vi "Untitled 2.vi"() -> ()   [LabVIEW 2014]
uses:
  Global 1.vi
panel:
  out "String":string
  in  "?":T1
  # "by Siavash Aghajani"
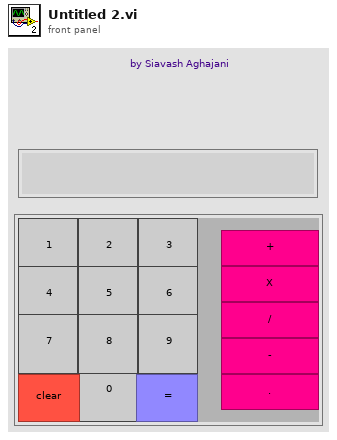
[diagram p1: front panel]
types:
  T1 = cluster{"Blank Button 2":bool, "Blank Button 3":bool, "Blank Button 4":bool, "Blank Button 5":bool, "Blank Button 6":bool, "Blank Button 7":bool, "Blank Button 8":bool, "Blank Button 9":bool, "Blank Button 10":bool, "Blank Button":bool, "Blank Button 11":bool, "Blank Button 12":bool, "Blank Button 13":bool, "Blank Button 14":bool, "Blank Button 15":bool, "Blank Button 16":bool, "OK Button":bool}
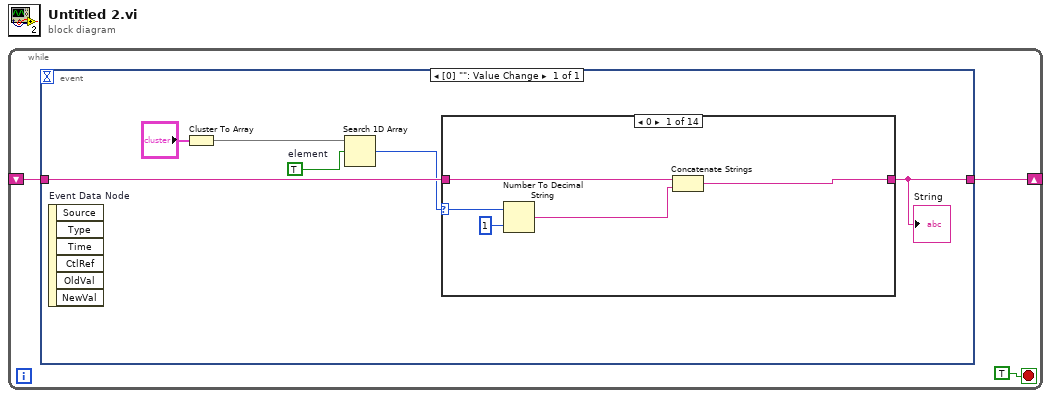
[diagram p0: block diagram]
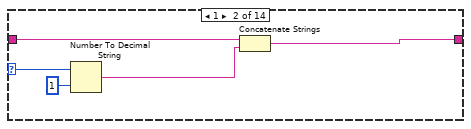
[diagram p2: hidden frame]
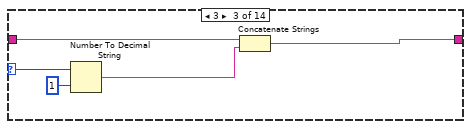
[diagram p3: hidden frame]
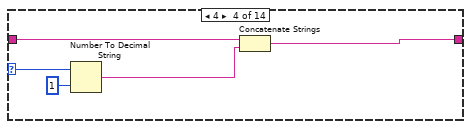
[diagram p4: hidden frame]
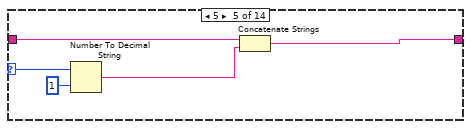
[diagram p5: hidden frame]
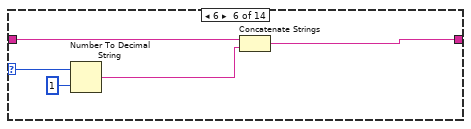
[diagram p6: hidden frame]
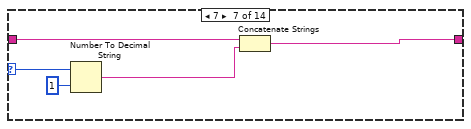
[diagram p7: hidden frame]
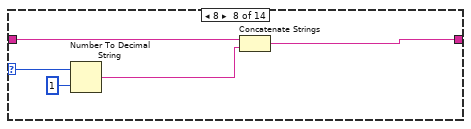
[diagram p8: hidden frame]
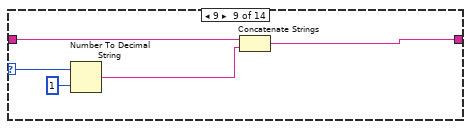
[diagram p9: hidden frame]
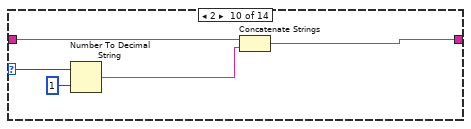
[diagram p10: hidden frame]
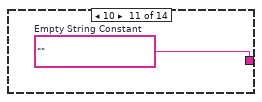
[diagram p11: hidden frame]
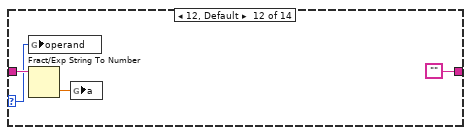
[diagram p12: hidden frame]
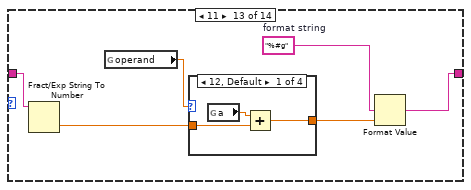
[diagram p13: hidden frame]
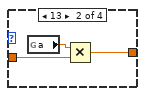
[diagram p14: hidden frame]
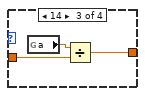
[diagram p15: hidden frame]
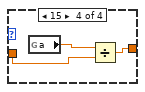
[diagram p16: hidden frame]
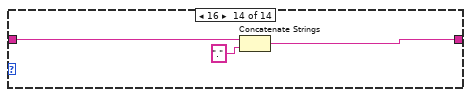
[diagram p17: hidden frame]
diagram:
  n1 = while {
    shift-right: [w1] -> _
    shift-left: _ -> [w2]
    stop <- TRUE stop-if-true
    n2 = event shown="[0] \"\": Value Change" {
      selector: _ -> [_]
      dyn-events: _ -> [_]
      timeout: _ -> [_]
      tunnel: w2 -> [w6]
      tunnel: [w5] -> w1
      event Value Change {
        w7 = TRUE  # element
        n3 = event-data "Event Data Node"() -> ()  [unwired: 1 in, 6 out]
        n4 = Cluster To Array(cluster="?") -> (array=w9:bool[])
        n5 = Search 1D Array(1D array=w9, element=w7) -> (index of element=w4:i32)  [unwired: 1 in]
        n6 = case shown="0" w4 {
          selector: w4 -> [w11 w16 w21 w26 w31 w36 w41 w46 w51 w56 _ w62 _ _]
          tunnel: w6 -> [w13 w18 w23 w28 w33 w38 w43 w48 w53 w58 _ w64 w69 w84]
          tunnel: [w12 w17 w22 w27 w32 w37 w42 w47 w52 w57 w60 "" w66 w85] -> w5
          frame 0 {
            n7 = Number To Decimal String(number=w11, width (-)=i16 1) -> (decimal integer string=w14:string)
            n8 = Concatenate Strings "Concatenate Strings"(w13, w14) -> (w12:string)
          }
          frame 1 {
            n9 = Number To Decimal String(number=w16, width (-)=i16 1) -> (decimal integer string=w19:string)
            n10 = Concatenate Strings "Concatenate Strings"(w18, w19) -> (w17:string)
          }
          frame 3 {
            n11 = Number To Decimal String(number=w21, width (-)=i16 1) -> (decimal integer string=w24:string)
            n12 = Concatenate Strings "Concatenate Strings"(w23, w24) -> (w22:string)
          }
          frame 4 {
            n13 = Number To Decimal String(number=w26, width (-)=i16 1) -> (decimal integer string=w29:string)
            n14 = Concatenate Strings "Concatenate Strings"(w28, w29) -> (w27:string)
          }
          frame 5 {
            n15 = Number To Decimal String(number=w31, width (-)=i16 1) -> (decimal integer string=w34:string)
            n16 = Concatenate Strings "Concatenate Strings"(w33, w34) -> (w32:string)
          }
          frame 6 {
            n17 = Number To Decimal String(number=w36, width (-)=i16 1) -> (decimal integer string=w39:string)
            n18 = Concatenate Strings "Concatenate Strings"(w38, w39) -> (w37:string)
          }
          frame 7 {
            n19 = Number To Decimal String(number=w41, width (-)=i16 1) -> (decimal integer string=w44:string)
            n20 = Concatenate Strings "Concatenate Strings"(w43, w44) -> (w42:string)
          }
          frame 8 {
            n21 = Number To Decimal String(number=w46, width (-)=i16 1) -> (decimal integer string=w49:string)
            n22 = Concatenate Strings "Concatenate Strings"(w48, w49) -> (w47:string)
          }
          frame 9 {
            n23 = Number To Decimal String(number=w51, width (-)=i16 1) -> (decimal integer string=w54:string)
            n24 = Concatenate Strings "Concatenate Strings"(w53, w54) -> (w52:string)
          }
          frame 2 {
            n25 = Number To Decimal String(number=w56, width (-)=i16 1) -> (decimal integer string=w59:string)
            n26 = Concatenate Strings "Concatenate Strings"(w58, w59) -> (w57:string)
          }
          frame 10 {
            w60 = ""  # Empty String Constant
          }
          frame 12, Default {
            n27 = global write "Global 1.vi" "operand"(w62) -> ()
            n28 = Fract/Exp String To Number(string=w64) -> (number=w61:dbl)  [unwired: 3 in, 1 out]
            n29 = global write "Global 1.vi" "a"(w61) -> ()
          }
          frame 11 {
            w67 = "%#g"  # format string
            n30 = Fract/Exp String To Number(string=w69) -> (number=w68:dbl)  [unwired: 3 in, 1 out]
            n31 = global read "Global 1.vi" "operand"() -> (w70:dbl)
            n32 = case shown="12, Default" w70 {
              tunnel: [w73 w76 w79 w82] -> w65
              tunnel: w68 -> [w71 w74 w77 w80]
              frame 12, Default {
                n33 = global read "Global 1.vi" "a"() -> (w72:dbl)
                n34 = Add(x=w72, y=w71) -> (x+y=w73:dbl)
              }
              frame 13 {
                n35 = global read "Global 1.vi" "a"() -> (w75:dbl)
                n36 = Multiply(x=w75, y=w74) -> (x*y=w76:dbl)
              }
              frame 14 {
                n37 = global read "Global 1.vi" "a"() -> (w78:dbl)
                n38 = Divide(x=w78, y=w77) -> (x/y=w79:dbl)
              }
              frame 15 {
                n39 = global read "Global 1.vi" "a"() -> (w81:dbl)
                n40 = Divide(x=w81, y=w80) -> (x/y=w82:dbl)
              }
            }
            n41 = Format Value(format string=w67, value (0)=w65) -> (output string=w66:string)  [unwired: 1 in]
          }
          frame 16 {
            n42 = Concatenate Strings "Concatenate Strings"(w84, ".") -> (w85:string)
          }
        }
        "String" <- w5
      }
    }
  }
